vi "Finish.vi"   [LabVIEW 2013]
doc: "This VI is called just before exiting. It is expected to close I/O refnum, save collected data, etc."
uses:
  <vilib>/Rock Robotics/WPI/Compressor/WPI_CompressorGetSetRefNum.vi
  <vilib>/Rock Robotics/WPI/Joystick/WPI_JoystickGetSetRefNum.vi
  <vilib>/Rock Robotics/WPI/RobotDrive/WPI_RobotDriveGetSetRefNum.vi
types:
  T1 = typedef "WPI_JoystickDevRef.ctl" = cluster{"Device":T2}
  T2 = typedef "WPI_JoystickDeviceEnum.ctl" = enum16{"USB 1", "USB 2", "USB 3", "USB 4", "Kinect 1", "Kinect 2"}
  T3 = typedef "WPI_RobotDriveDevRef.ctl" = cluster{"DevStatus":errorcluster, "Motors[]":T4[], "Square Inputs":bool, "Max Output":dbl, "Isochronous":bool}
  T4 = typedef "WPI_MotorControlDeviceRef.ctl" = cluster{"DeviceStatus":errorcluster, "Type":enum16{"PWM", "CAN"}, "PWM":cluster{"Digital Module":T5, "PWM Channel":T6, "DeadBand":T7}, "CAN":cluster{"Device Number":u8, "Control Mode":T8, "Semaphore":T9, "Max Vout":dbl}, "Invert":bool, "TransformRef":T10, "InvTransformRef":T10}
  T5 = typedef "FPGA_TypedefDigitalModule.ctl" = enum16{"Digital Module 1", "Digital Module 2"}
  T6 = typedef "FPGA_DIOPWMChannel.ctl" = enum8{"PWM 1", "PWM 2", "PWM 3", "PWM 4", "PWM 5", "PWM 6", "PWM 7", "PWM 8", "PWM 9", "PWM 10", "Invalid"}
  T7 = typedef "WPI_PWMDeadband.ctl" = cluster{"Name":string, "maxPositivePwm":i32, "minPositivePwm":i32, "centerPwm":i32, "maxNegativePwm":i32, "minNegativePwm":i32, "angularRange":u16}
  T8 = typedef "WPI_CANJaguar_ControlMode.ctl" = enum8{"Percent VBus", "Current", "Speed", "Position", "Voltage"}
  T9 = typedef "Semaphore RefNum" = refnum<k1>
  T10 = typedef "WPI_PWMTransform_ConPane.ctl" = refnum<vi>
  T11 = typedef "WPI_ServoDeviceRef.ctl" = cluster{"DeviceStatus":errorcluster, "Digital Module":T5, "PWM Channel":T6, "DeadBand":T7}
  T12 = typedef "WPI_SolenoidDevRef.ctl" = cluster{"DevStatus":errorcluster, "Solenoid Module":T13, "Forward Solenoid Channel":T14, "Reverse Solenoid Channel":T14}
  T13 = typedef "FPGA_TypedefSolenoidModule.ctl" = enum16{"Solenoid Module 1", "Solenoid Module 2"}
  T14 = typedef "WPI_SolenoidChannel.ctl" = enum8{"Solenoid 1", "Solenoid 2", "Solenoid 3", "Solenoid 4", "Solenoid 5", "Solenoid 6", "Solenoid 7", "Solenoid 8", "Invalid"}
  T15 = typedef "WPI_DigitalInputDevRef.ctl" = cluster{"DevStatus":errorcluster, "DIO Channel":T16, "Digital Module":T5}
  T16 = typedef "FPGA_DIOChannel.ctl" = enum8{"DIO 1", "DIO 2", "DIO 3", "DIO 4", "DIO 5", "DIO 6", "DIO 7", "DIO 8", "DIO 9", "DIO 10", "DIO 11", "DIO 12", "DIO 13", "DIO 14", "Invalid"}
  T17 = typedef "WPI_CompressorDevRef.ctl" = cluster{"DevStatus":errorcluster, "DigitalInputDevRef":T15, "RelayDevRef":T18}
  T18 = typedef "WPI_RelayDevRef.ctl" = cluster{"DevStatus":errorcluster, "Relay Channel":T19, "Digital Module":T5, "Relay Direction":T20}
  T19 = typedef "FPGA_DIORelayChannel.ctl" = enum8{"Relay 1", "Relay 2", "Relay 3", "Relay 4", "Relay 5", "Relay 6", "Relay 7", "Relay 8", "Invalid"}
  T20 = typedef "WPI_RelayDirection.ctl" = enum16{"Both directions", "Forward only", "Reverse only"}
  T21 = typedef "WPI_GyroDevRef.ctl" = cluster{"DevStatus":errorcluster, "Analog Module":T22, "Analog Channel":T23, "Offset":dbl, "Gain (VoltsPerDegree/Second)":dbl}
  T22 = typedef "FPGA_TypedefAnalogModule.ctl" = enum16{"Analog Module 1", "Analog Module 2"}
  T23 = typedef "FPGA_AIChannel.ctl" = enum8{"AI 1", "AI 2", "AI 3", "AI 4", "AI 5", "AI 6", "AI 7", "AI 8", "Invalid"}
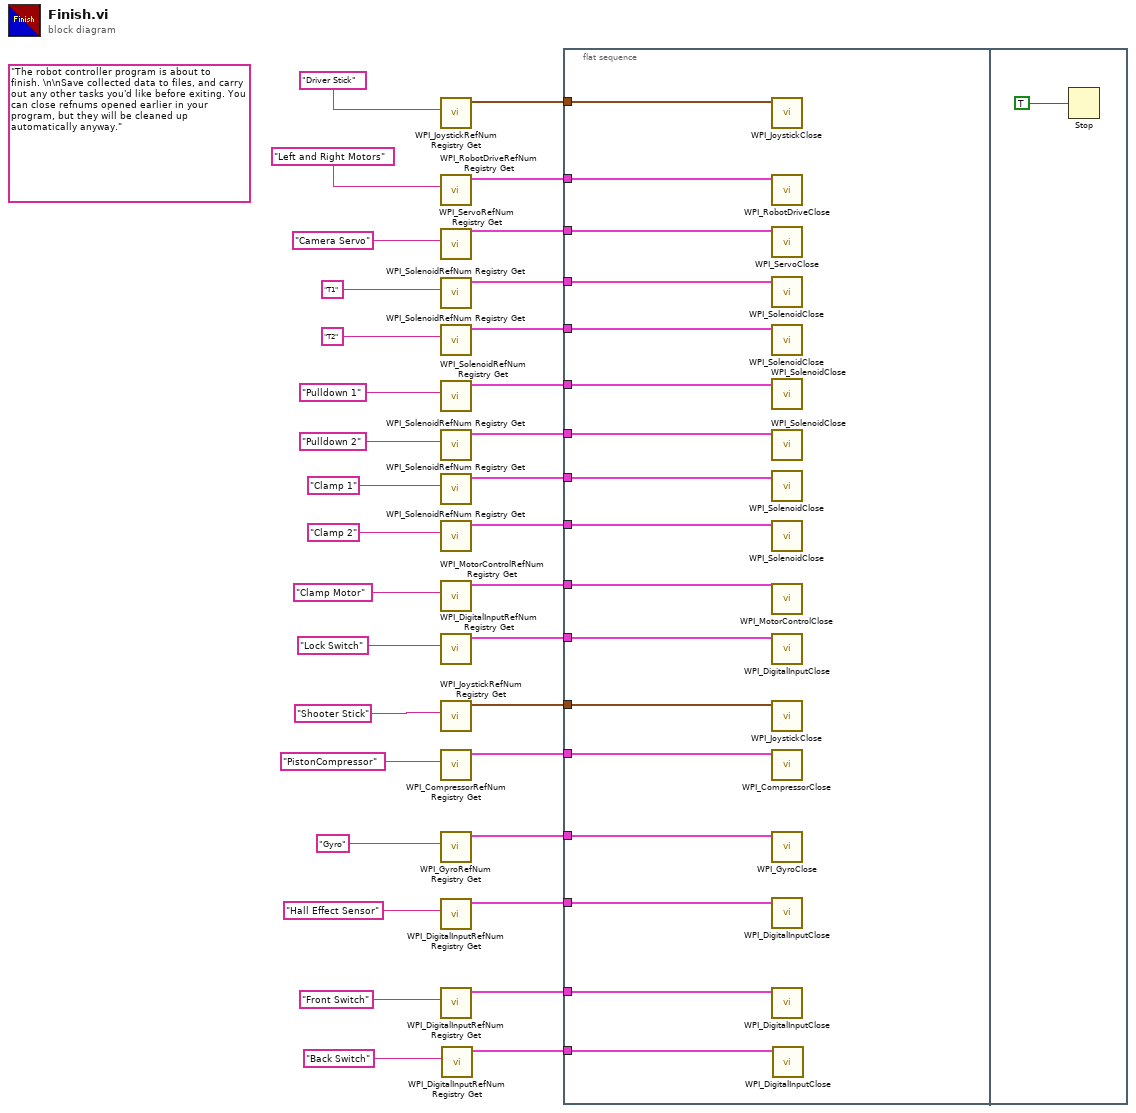
[diagram p0: block diagram]
diagram:
  (unwired) "The robot controller program is about to finish. \n\nSave collected data to files, and carry out any other tasks you'd like before exiting. You can close refnums opened earlier in your program, but they will be cleaned up automatically anyway."
  n1 = call <vilib>:"WPI_JoystickRefNum Registry Get.vi"("refnum name"="Driver Stick") -> ("JoystickDevRef"=w31:T1)  [unwired: 1 in, 9 out]
  n2 = call <vilib>:"WPI_RobotDriveRefNum Registry Get.vi"("refnum name"="Left and Right Motors") -> ("RobotDriveDevRef"=w32:T3)  [unwired: 1 in, 9 out]
  n3 = call <vilib>:"WPI_ServoRefNum Registry Get.vi"("refnum name"="Camera Servo") -> ("ServoDeviceRef"=w29:T11)  [unwired: 9 in, 1 out]
  n4 = call <vilib>:"WPI_SolenoidRefNum Registry Get.vi"("refnum name"="T1") -> ("SolenoidDevRef"=w28:T12)  [unwired: 9 in, 1 out]
  n5 = call <vilib>:"WPI_SolenoidRefNum Registry Get.vi"("refnum name"="T2") -> ("SolenoidDevRef"=w21:T12)  [unwired: 9 in, 1 out]
  n6 = call <vilib>:"WPI_SolenoidRefNum Registry Get.vi"("refnum name"="Pulldown 1") -> ("SolenoidDevRef"=w20:T12)  [unwired: 9 in, 1 out]
  n7 = call <vilib>:"WPI_SolenoidRefNum Registry Get.vi"("refnum name"="Pulldown 2") -> ("SolenoidDevRef"=w19:T12)  [unwired: 9 in, 1 out]
  n8 = call <vilib>:"WPI_SolenoidRefNum Registry Get.vi"("refnum name"="Clamp 1") -> ("SolenoidDevRef"=w18:T12)  [unwired: 9 in, 1 out]
  n9 = call <vilib>:"WPI_SolenoidRefNum Registry Get.vi"("refnum name"="Clamp 2") -> ("SolenoidDevRef"=w17:T12)  [unwired: 9 in, 1 out]
  n10 = call <vilib>:"WPI_MotorControlRefNum Registry Get.vi"("refnum name"="Clamp Motor") -> ("MotorControlDevRef"=w16:T4)  [unwired: 9 in, 1 out]
  n11 = call <vilib>:"WPI_DigitalInputRefNum Registry Get.vi"("refnum name"="Lock Switch") -> ("DigitalInputDevRef"=w13:T15)  [unwired: 9 in, 1 out]
  n12 = call <vilib>:"WPI_JoystickRefNum Registry Get.vi"("refnum name"="Shooter Stick") -> ("JoystickDevRef"=w12:T1)  [unwired: 1 in, 9 out]
  n13 = call <vilib>:"WPI_CompressorRefNum Registry Get.vi"("refnum name"="PistonCompressor") -> ("CompressorDevRef"=w9:T17)  [unwired: 9 in, 1 out]
  n14 = call <vilib>:"WPI_GyroRefNum Registry Get.vi"("refnum name"="Gyro") -> ("GyroDevRef"=w8:T21)  [unwired: 9 in, 1 out]
  n15 = call <vilib>:"WPI_DigitalInputRefNum Registry Get.vi"("refnum name"="Hall Effect Sensor") -> ("DigitalInputDevRef"=w5:T15)  [unwired: 9 in, 1 out]
  n16 = call <vilib>:"WPI_DigitalInputRefNum Registry Get.vi"("refnum name"="Front Switch") -> ("DigitalInputDevRef"=w4:T15)  [unwired: 9 in, 1 out]
  n17 = call <vilib>:"WPI_DigitalInputRefNum Registry Get.vi"("refnum name"="Back Switch") -> ("DigitalInputDevRef"=w1:T15)  [unwired: 9 in, 1 out]
  n18 = flat-sequence {
    tunnel: w32 -> [w51]
    tunnel: w31 -> [w50]
    tunnel: w29 -> [w49]
    tunnel: w28 -> [w48]
    tunnel: w21 -> [w47]
    tunnel: w20 -> [w46]
    tunnel: w19 -> [w45]
    tunnel: w18 -> [w44]
    tunnel: w17 -> [w43]
    tunnel: w16 -> [w42]
    tunnel: w13 -> [w41]
    tunnel: w12 -> [w40]
    tunnel: w9 -> [w39]
    tunnel: w8 -> [w38]
    tunnel: w5 -> [w37]
    tunnel: w4 -> [w36]
    tunnel: w1 -> [w35]
    frame #0 {
      n19 = call <vilib>:"WPI_JoystickClose.vi"("JoystickDevRef"=w50) -> ()  [unwired: 11 out]
      n20 = call <vilib>:"WPI_RobotDriveClose.vi"("RobotDriveDevRef"=w51) -> ()  [unwired: 1 in, 10 out]
      n21 = call <vilib>:"WPI_ServoClose.vi"("MotorControlDevRef"=w49) -> ()  [unwired: 10 in, 1 out]
      n22 = call <vilib>:"WPI_SolenoidClose.vi"("SolenoidDevRef"=w48) -> ()  [unwired: 10 in, 1 out]
      n23 = call <vilib>:"WPI_SolenoidClose.vi"("SolenoidDevRef"=w47) -> ()  [unwired: 10 in, 1 out]
      n24 = call <vilib>:"WPI_SolenoidClose.vi"("SolenoidDevRef"=w46) -> ()  [unwired: 10 in, 1 out]
      n25 = call <vilib>:"WPI_SolenoidClose.vi"("SolenoidDevRef"=w45) -> ()  [unwired: 10 in, 1 out]
      n26 = call <vilib>:"WPI_SolenoidClose.vi"("SolenoidDevRef"=w44) -> ()  [unwired: 10 in, 1 out]
      n27 = call <vilib>:"WPI_SolenoidClose.vi"("SolenoidDevRef"=w43) -> ()  [unwired: 10 in, 1 out]
      n28 = call <vilib>:"WPI_MotorControlClose.vi"("MotorControlDevRef"=w42) -> ()  [unwired: 10 in, 1 out]
      n29 = call <vilib>:"WPI_DigitalInputClose.vi"("DigitalInputDevRef"=w41) -> ()  [unwired: 10 in, 1 out]
      n30 = call <vilib>:"WPI_JoystickClose.vi"("JoystickDevRef"=w40) -> ()  [unwired: 11 out]
      n31 = call <vilib>:"WPI_CompressorClose.vi"("CompressorDevRef"=w39) -> ()  [unwired: 10 in, 1 out]
      n32 = call <vilib>:"WPI_GyroClose.vi"("GyroDevRef"=w38) -> ()  [unwired: 1 in, 10 out]
      n33 = call <vilib>:"WPI_DigitalInputClose.vi"("DigitalInputDevRef"=w37) -> ()  [unwired: 10 in, 1 out]
      n34 = call <vilib>:"WPI_DigitalInputClose.vi"("DigitalInputDevRef"=w36) -> ()  [unwired: 10 in, 1 out]
      n35 = call <vilib>:"WPI_DigitalInputClose.vi"("DigitalInputDevRef"=w35) -> ()  [unwired: 10 in, 1 out]
    }
    frame #1 {
      n36 = Stop(stop? (T)=TRUE ("Quit")) -> ()
    }
  }
